vi "PlugIn Relay.vi"(6 "String Value":string, 10 "Channel":T2, 11 "Menu":T1=enum."set init_rev") -> ()   [LabVIEW 2019]
uses:
  Relay Update Ops.ctl
  <vilib>/Rock Robotics/SystemInterfaces/DIO/FPGA_DIORelayChannel.ctl
panel:
  # "Don't place this VI anywhere\nin your API code. It needs to\nbe a dynamically loaded\nwrapper of the main global"
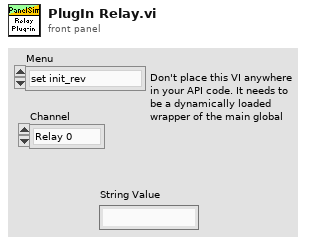
[diagram p1: front panel]
types:
  T1 = typedef "Relay Update Ops.ctl" = enum16{"set init_fwd", "set init_rev", "set fwd", "set rev", "get", "delete", "JSON update", "set name", "transmit initial", "reset"}
  T2 = typedef "FPGA_DIORelayChannel.ctl" = enum8{"Relay 0", "Relay 1", "Relay 2", "Relay 3", "Invalid"}
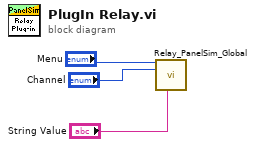
[diagram p0: block diagram]
diagram:
  n1 = call "Relay_PanelSim_Global.vi"("menu"="Menu", "RelayChannel"="Channel", "String Value"="String Value") -> ()  [unwired: 11 in, 2 out]
